vi "colourDilute.vi"(6 "dilutionFactor":dbl=0.5000000000000001 min=0.0 max=1.0 step=0.1, 11 "RGBIn":cluster{"R":sgl, "G":sgl, "B":sgl, "A":sgl}) -> (2 "colourOut":u32(colorbox), 3 "RGBOut":cluster{"R":dbl, "G":dbl, "B":dbl, "A":dbl})   [LabVIEW 2022 SP3]
panel:
  out "colourIn":u32(colorbox)
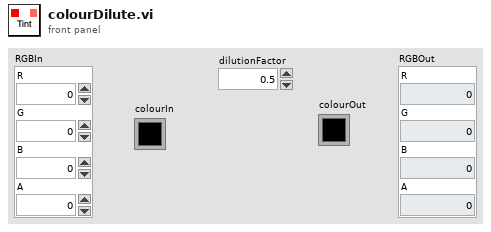
[diagram p1: front panel]
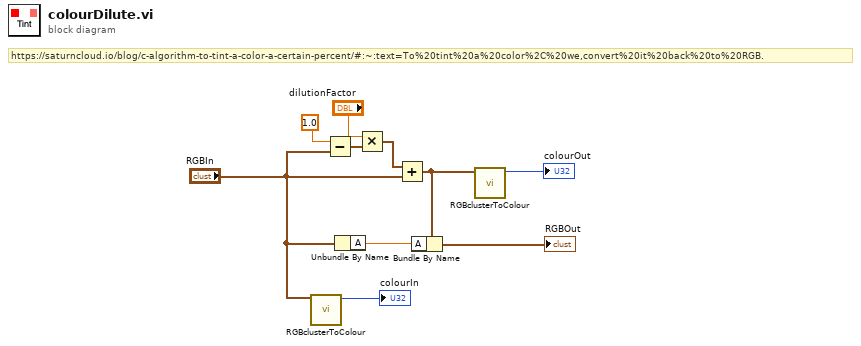
[diagram p0: block diagram]
diagram:
  # "https://saturncloud.io/blog/c-algorithm-to-tint-a-color-a-certain-percent/#:~:text=To%20tint%20a%20color%2C%20we,convert%20it%20back%20to%20RGB."
  n1 = call "RGBclusterToColour.vi"("RGBin"="RGBIn") -> ("colour"=→"colourIn":u32)  [unwired: 10 in]
  n2 = Subtract(x=1.0, y="RGBIn") -> (x-y=w5:cluster{"R":dbl, "G":dbl, "B":dbl, "A":dbl})
  n3 = Unbundle By Name("RGBIn") -> ("A"=w9:sgl)
  n4 = Multiply(x="dilutionFactor", y=w5) -> (x*y=w3:cluster{"R":dbl, "G":dbl, "B":dbl, "A":dbl})
  n5 = Add(x=w3, y="RGBIn") -> (x+y=w1:cluster{"R":dbl, "G":dbl, "B":dbl, "A":dbl})
  n6 = Bundle By Name(cluster=w1, "A"=w9) -> (→"RGBOut":cluster{"R":dbl, "G":dbl, "B":dbl, "A":dbl})
  n7 = call "RGBclusterToColour.vi"("RGBin"=w1) -> ("colour"=→"colourOut":u32)  [unwired: 10 in]
